vi "num2lett.vi"(1 "Number":i32) -> (0 "LetterCombination":string)   [LabVIEW 2018]
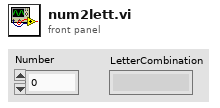
[diagram p1: front panel]
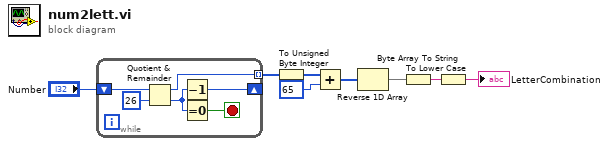
[diagram p0: block diagram]
diagram:
  n1 = while {
    tunnel: [w13] -> w8 mode=indexing
    shift-right: [w9] -> _
    shift-left: "Number" -> [w14]
    stop <- w12 stop-if-true
    n2 = Quotient & Remainder(x=w14, y=26) -> (x-y*floor(x/y)=w13:i32, floor(x/y)=w11:i32)
    n3 = Decrement(x=w11) -> (x-1=w9:i32)
    n4 = Equal To 0?(x=w11) -> (x = 0?=w12:bool)
  }
  n5 = To Unsigned Byte Integer(number=w8) -> (unsigned 8bit integer=w4:u8[])
  n6 = Add(x=w4, y=u8 65) -> (x+y=w6:u8[])
  n7 = Reverse 1D Array(array=w6) -> (reversed array=w7:u8[])
  n8 = Byte Array To String(unsigned byte array=w7) -> (string=w2:string)
  n9 = To Lower Case(string=w2) -> (all lower case string=→"LetterCombination":string)
